vi "Custom Z Sweep (pt by pt).vi"() -> ()   [LabVIEW 2016]
doc: "This example performs a custom Z sweep.\n\n- Nanonis Programming Interface -"
uses:
  Nanonis Prog Interface.lvlib
panel:
  in  "Settling time (ms)":u32=20 max=10000
  out "Steps done":i32=99
  out "XY Graph":cluster{sgl[], "Signals Values":sgl[]}(graph)
  in  "Stop":bool
  in  "Sweep distance (m)":sgl=1e-09 min=-1e-07 max=1e-07 format="%#_5p"
  in  "N points":i32=100 min=2 max=10000
  # "Example program for the Nanonis SPM Control software programming interface\n\n - Custom Z Sweep -"
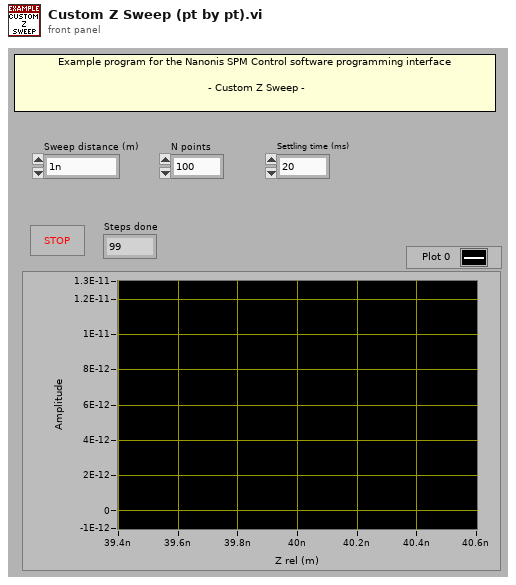
[diagram p1: front panel]
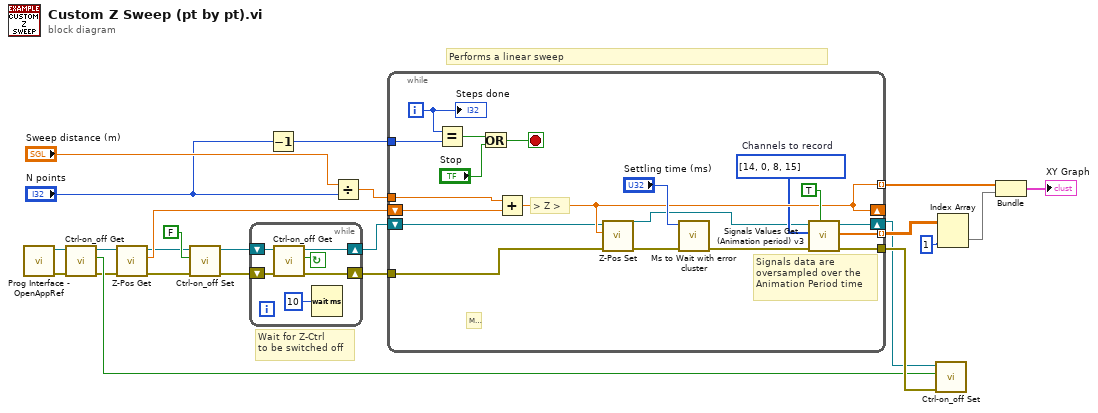
[diagram p0: block diagram]
diagram:
  # "Performs a linear sweep"
  # "Missing object. The object Loop Condition does not exist in the previous version."
  # "Wait for Z-Ctrl\nto be switched off"
  n1 = call <userlib>:"Prog Interface - OpenAppRef.vi"() -> ("Error out"=w18:errorcluster, "Application reference"=w8:refnum<vi>)  [unwired: 6 in]
  n2 = call <userlib>:"Ctrl-on_off Get.vi"("error in (no error)"=w18, "Application ref in"=w8) -> ("error out"=w13:errorcluster, "Z-Controller on/off status"=w14:bool, "Application ref out"=w7:refnum<vi>)  [unwired: 7 in]
  n3 = call <userlib>:"Z-Pos Get.vi"("error in (no error)"=w13, "Application ref in"=w7) -> ("error out"=w12:errorcluster, "Z position (m)"=w11:sgl, "Application ref out"=w6:refnum<vi>)  [unwired: 7 in]
  n4 = call <userlib>:"Ctrl-on_off Set.vi"("error in (no error)"=w12, "Z Controller ON/OFF"=FALSE, "Application ref in"=w6) -> ("error out"=w10:errorcluster, "Application ref out"=w5:refnum<vi>)  [unwired: 7 in]
  n5 = while {
    shift-right: [w30] -> w9
    shift-left: w10 -> [w29]
    shift-right: [w25] -> w4
    shift-left: w5 -> [w26]
    stop <- w28 continue-if-true
    n6 = call <userlib>:"Ctrl-on_off Get.vi"("error in (no error)"=w29, "Application ref in"=w26) -> ("error out"=w30:errorcluster, "Z-Controller on/off status"=w28:bool, "Application ref out"=w25:refnum<vi>)  [unwired: 7 in]
    n7 = Wait (ms)(milliseconds to wait=u32 10) -> ()  [unwired: 1 out]
  }
  n8 = Decrement(x="N points") -> (x-1=w1:i32)
  n9 = Divide(x="Sweep distance (m)", y="N points") -> (x/y=w19:sgl)
  n10 = while {
    tunnel: w9 -> [w43]
    tunnel: [w49] -> w16
    tunnel: [w35] -> w24 mode=indexing
    shift-right: [w37] -> _
    shift-left: w11 -> [w47]
    tunnel: w19 -> [w48]
    tunnel: [w37] -> w15 mode=indexing
    tunnel: w1 -> [w31]
    shift-right: [w34] -> w3
    shift-left: w4 -> [w36]
    i -> [w41]
    stop <- w39 stop-if-true
    w33 = i8[] [14, 0, 8, 15]  # Channels to record
    # "Signals data are \noversampled over the \nAnimation Period time"
    # "> Z >"
    n11 = Equal?(x=w41, y=w31) -> (x = y?=w40:bool)
    n12 = Or(x=w40, y="Stop") -> (x .or. y?=w39:bool)
    n13 = Add(x=w48, y=w47) -> (x+y=w37:sgl)
    n14 = call <userlib>:"Z-Pos Set.vi"("error in (no error)"=w43, "Z position (m)"=w37, "Application ref in"=w36) -> ("error out"=w46:errorcluster, "Application ref out"=w32:refnum<vi>)  [unwired: 7 in]
    n15 = call "Ms to Wait with error cluster.vi"("error in (no error)"=w46, "milliseconds to wait"="Settling time (ms)") -> ("error out"=w45:errorcluster)  [unwired: 4 in, 1 out]
    n16 = call <userlib>:"Signals Values Get (Animation period) v3.vi"("Wait for newest data (F=False)"=TRUE ("Wait for newest data (F)"), "error in (no error)"=w45, "Signals indexes (0-127)"=w33, "Application ref in"=w32) -> ("error out"=w49:errorcluster, "Signals Values"=w35:sgl[], "Application ref out"=w34:refnum<vi>)  [unwired: 4 in]
    "Steps done" <- w41
  }
  n17 = call <userlib>:"Ctrl-on_off Set.vi"("error in (no error)"=w16, "Z Controller ON/OFF"=w14, "Application ref in"=w3) -> ()  [unwired: 7 in, 2 out]
  n18 = Index Array(array=w24, index (col)=1 ("disabled index (col)")) -> (element=w22:sgl[])  [unwired: 1 in]
  n19 = Bundle(w15, "Signals Values"=w22) -> (→"XY Graph":cluster{sgl[], "Signals Values":sgl[]})  [unwired: 1 in]
